vi "Arm Up.vi"() -> ()   [LabVIEW 2015]
uses:
  References/Refnums.vi
  <vilib>/ptbypt/NI_PtbyPt.lvlib
panel:
  in  "error in":errorcluster
  out "error out":errorcluster
  in  "Time":dbl
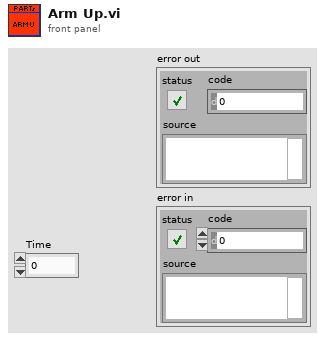
[diagram p1: front panel]
types:
  T1 = typedef "WPI_MotorControlDeviceRef.ctl" = cluster{"DeviceStatus":errorcluster, "Type":T2, "PWM":cluster{"PWM Channel":T3, "DeadBand":T4}, "CAN":cluster{"Device Number":u8, "Control Mode":T5, "Semaphore":T6, "Max Vout":dbl, "TalonSRX Control Mode":T7}, "Invert":bool}
  T2 = typedef "WPI_MotorControlType.ctl" = enum16{"PWM", "CAN", "CANTalonSRX"}
  T3 = typedef "FPGA_DIOPWMChannel.ctl" = enum8{"PWM 0", "PWM 1", "PWM 2", "PWM 3", "PWM 4", "PWM 5", "PWM 6", "PWM 7", "PWM 8", "PWM 9", "PWM MXP 0", "PWM MXP 1", "PWM MXP 2", "PWM MXP 3", "PWM MXP 4", "PWM MXP 5", "PWM MXP 6", "PWM MXP 7", "PWM MXP 8", "PWM MXP 9", "Invalid"}
  T4 = typedef "WPI_PWMDeadband.ctl" = cluster{"Name":string, "maxPositivePwm":i32, "minPositivePwm":i32, "centerPwm":i32, "maxNegativePwm":i32, "minNegativePwm":i32, "angularRange":u16}
  T5 = typedef "WPI_CANJaguar_ControlMode.ctl" = enum8{"Percent VBus", "Current", "Speed", "Position", "Voltage"}
  T6 = typedef "Semaphore RefNum" = refnum<k1>
  T7 = typedef "WPI_CANTalonSRX_APIControlMode.ctl" = enum8{"Percent VBus", "Speed", "Position", "Slave", "Unchanged / Invalid", "Voltage Compensation", "Current", "Motion Profile"}
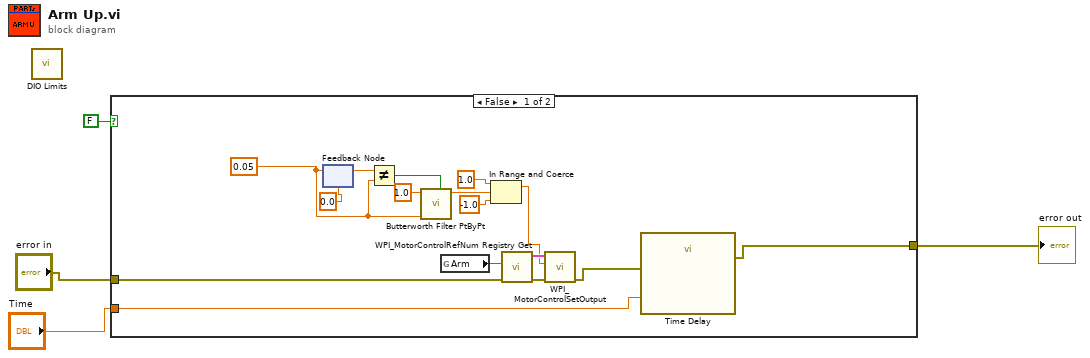
[diagram p0: block diagram]
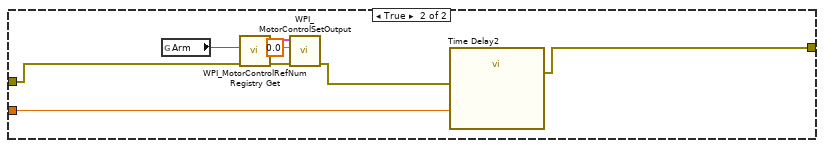
[diagram p2: hidden frame]
diagram:
  n1 = call "DIO Limits.vi"() -> ()  [unwired: 10 in, 2 out]
  n2 = case shown="False" FALSE {
    tunnel: "error in" -> [w8 w24]
    tunnel: [w7 w21] -> w2
    tunnel: "Time" -> [w6 w23]
    frame False {
      w17 = 0.05 ("Low Pass Filter Average Length")
      n3 = feedback #1(0.0 ("Low Pass Filter Average Length")) -> (w14:dbl)
      n4 = feedback-in #1(w17) -> ()
      n5 = Not Equal?(x=w14, y=w17) -> (x != y?=w15:bool)
      n6 = call <vilib>:"Butterworth Filter PtByPt.vi"("initialize"=w15, "low cutoff freq: fl"=w17, "x"=1.0) -> ("Filtered x"=w11:dbl)  [unwired: 6 in, 1 out]
      n7 = global read "Refnums.vi" "Arm"() -> (w20:string)
      n8 = In Range and Coerce(upper limit=1.0, x=w11, lower limit=-1.0) -> (coerced(x)=w10:dbl)  [unwired: 1 out]
      n9 = call <vilib>:"WPI_MotorControlRefNum Registry Get.vi"("error in (no error)"=w8, "refnum name"=w20) -> ("error out"=w18:errorcluster, "MotorControlDevRef"=w19:T1)  [unwired: 8 in]
      n10 = call <vilib>:"WPI_MotorControlSetOutput.vi"("error in (no error)"=w18, "Output"=w10, "MotorControlDevRef"=w19) -> ("error out"=w9:errorcluster)  [unwired: 6 in, 2 out]
      n11 = call "Time Delay"("error in (no error)"=w9, "Delay Time (s)"=w6) -> ("error out"=w7:errorcluster)  [unwired: 9 in]
    }
    frame True {
      n12 = global read "Refnums.vi" "Arm"() -> (w28:string)
      n13 = call <vilib>:"WPI_MotorControlRefNum Registry Get.vi"("error in (no error)"=w24, "refnum name"=w28) -> ("error out"=w26:errorcluster, "MotorControlDevRef"=w27:T1)  [unwired: 8 in]
      n14 = call <vilib>:"WPI_MotorControlSetOutput.vi"("error in (no error)"=w26, "Output"=0.0, "MotorControlDevRef"=w27) -> ("error out"=w22:errorcluster)  [unwired: 6 in, 2 out]
      n15 = call "Time Delay2"("error in (no error)"=w22, "Delay Time (s)"=w23) -> ("error out"=w21:errorcluster)  [unwired: 9 in]
    }
  }
  "error out" <- w2
